vi "Query.vi"(8 "error in":errorcluster, 10 "Query":string, 11 "DB-SQLite in":refnum<class "DB-SQLite.lvclass">) -> (0 "error out":errorcluster, 1 "Meta Data":variant, 2 "Return Data":string[][](table) caption="Result Set (from first statement with results)", 3 "DB-SQLite out":refnum<class "DB-SQLite.lvclass">, 4 "Field Names":string[](array[string]))   [LabVIEW 2020, in "hse-db-sqlite.lvlib" / "DB-SQLite.lvclass"]
doc: "____\nHAMPEL SOFTWARE ENGINEERING v1.4.0 (2023-12-19 09:52)"
uses:
  DB-SQLite.lvclass
  DB-SQLite.lvclass/DB-SQLite.ctl
  <vilib>/drjdpowell/SQLite Library/SQL Connection/Execute SQL.vi
  <vilib>/drjdpowell/SQLite Library/SQLite.lvlib
  <vilib>/drjdpowell/SQLite Library/SQL Connection/Connection.lvclass
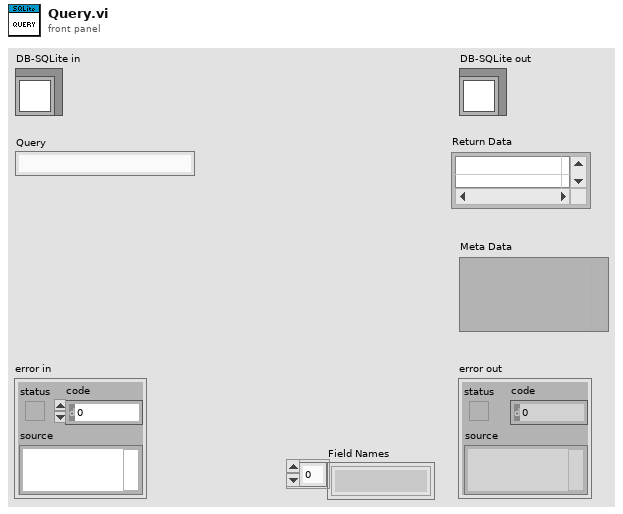
[diagram p1: front panel]
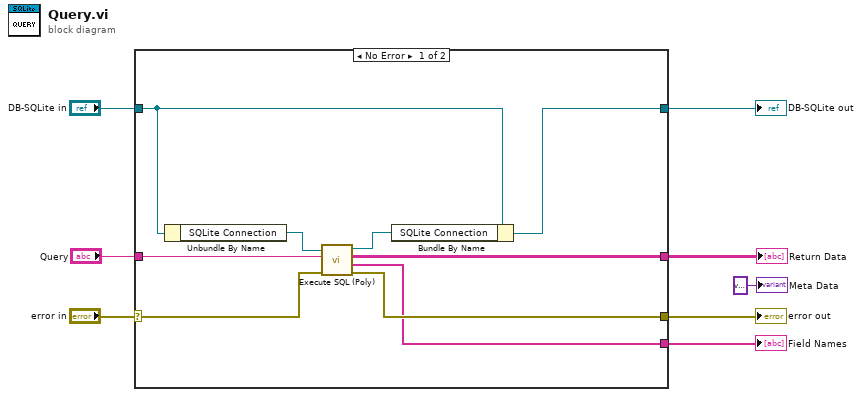
[diagram p0: block diagram]
diagram:
  n1 = case shown="No Error" "error in" {
    selector: "error in" -> [w17 w19]
    tunnel: [w16 w19] -> w7
    tunnel: [w12 w18] -> w5
    tunnel: "DB-SQLite in" -> [w13 w18]
    tunnel: "Query" -> [w15 _]
    tunnel: [w10 _] -> w3
    tunnel: [w9 _] -> w2
    frame No Error {
      n2 = Unbundle By Name(w13) -> ("SQLite Connection"=w14:refnum<class "Connection.lvclass">)
      n3 = call-poly <vilib>:"Execute SQL (Poly).vi"("error in (no error)"=w17, "SQL"=w15, "SQLite Connection in"=w14) -> ("error out"=w16:errorcluster, "Column Names"=w9:string[], "Result Set"=w10:string[][], "SQLite Connection"=w11:refnum<class "Connection.lvclass">)  [unwired: 5 in]
      n4 = Bundle By Name(cluster=w13, "SQLite Connection"=w11) -> (w12:refnum<class "DB-SQLite.lvclass">)
    }
    frame Error {
    }
  }
  "error out" <- w7
  "DB-SQLite out" <- w5
  "Return Data" <- w3
  "Field Names" <- w2
  "Meta Data" <- variant ("Meta Data")
